vi "check if file name already exists.vi"(8 "error in (no error)":errorcluster, 9 "file to write":path, 10 "Folder Path":path, 11 "DAQOrcaFlash in":refnum<class "DAQOrcaFlash.lvclass">) -> (0 "error out":errorcluster, 1 "file to write":path, 2 "file exists?":bool, 3 "DAQOrcaFlash out":refnum<class "DAQOrcaFlash.lvclass">)   [LabVIEW 2012, in "DAQOrcaFlash.lvclass"]
uses:
  DAQOrcaFlash.lvclass
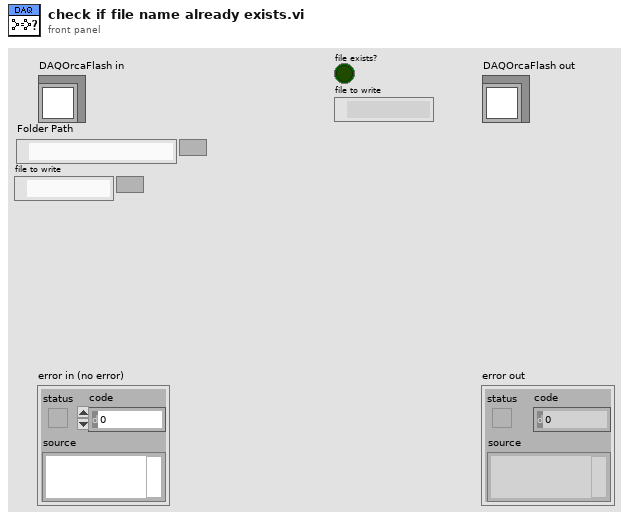
[diagram p1: front panel]
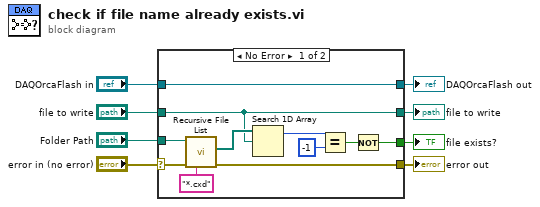
[diagram p0: block diagram]
diagram:
  n1 = case shown="No Error" "error in (no error)" {
    selector: "error in (no error)" -> [w10 w21]
    tunnel: [w9 w21] -> w7
    tunnel: [w19 w20] -> w5
    tunnel: "DAQOrcaFlash in" -> [w19 w20]
    tunnel: "Folder Path" -> [w18 _]
    tunnel: "file to write" -> [w11 _]
    tunnel: [w12 _] -> w2
    tunnel: [w11 _] -> w1
    frame No Error {
      n2 = call <vilib>:"Recursive File List.vi"("pattern"="*.cxd", "error in (no error)"=w10, "Folder Path"=w18) -> ("error out"=w9:errorcluster, "All Files in Dir"=w16:path[])  [unwired: 4 in, 3 out]
      n3 = Search 1D Array(1D array=w16, element=w11) -> (index of element=w15:i32)  [unwired: 1 in]
      n4 = Equal?(x=w15, y=-1) -> (x = y?=w13:bool)
      n5 = Not(x=w13) -> (.not. x?=w12:bool)
    }
    frame Error {
    }
  }
  "error out" <- w7
  "DAQOrcaFlash out" <- w5
  "file exists?" <- w2
  "file to write" <- w1
